vi "Apply_Rect_Offset.vi"(3 "do offset":bool=TRUE, 4 "offset rect":T1, 5 "input":T1) -> (2 "output":T1)   [LabVIEW 2012]
uses:
  <userlib>/BIAS2/subvis/ROI_rect.ctl
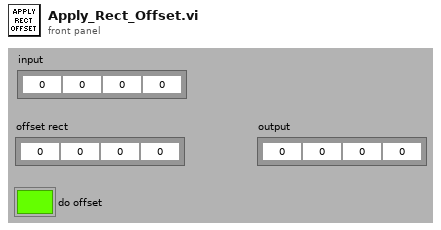
[diagram p1: front panel]
types:
  T1 = typedef "ROI_rect.ctl" = cluster{"left":i32, "top":i32, "right":i32, "bottom":i32}
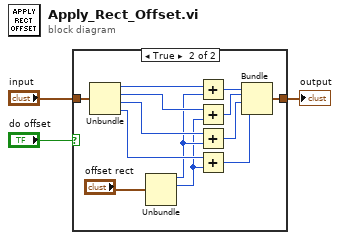
[diagram p0: block diagram]
diagram:
  n1 = case shown="True" "do offset" {
    tunnel: "input" -> [w4 w17]
    tunnel: [w4 w11] -> w1
    frame False {
    }
    frame True {
      n2 = Unbundle(w17) -> ("left"=w10:i32, "top"=w9:i32, "right"=w8:i32, "bottom"=w7:i32)
      n3 = Unbundle("offset rect") -> ("left"=w6:i32, "top"=w5:i32)  [unwired: 2 out]
      n4 = Add(x=w10, y=w6) -> (x+y=w15:i32)
      n5 = Add(x=w9, y=w5) -> (x+y=w14:i32)
      n6 = Add(x=w8, y=w6) -> (x+y=w13:i32)
      n7 = Add(x=w7, y=w5) -> (x+y=w12:i32)
      n8 = Bundle(w15, w14, w13, w12) -> (w11:cluster{i32, i32, i32, i32})  [unwired: 1 in]
    }
  }
  "output" <- w1
